vi "Drag Start Row Visualization.vi"(7 "DragStart? (F)":bool, 8 "error in (no error)":errorcluster, 10 "DragStart Indices":i32[](array[numeric]), 11 "BetterListboxHandle in":refnum<class "BetterListboxHandle.lvclass">) -> (0 "error out":errorcluster, 3 "BetterListboxHandle out":refnum<class "BetterListboxHandle.lvclass">)   [LabVIEW 2020, in "BetterDragAndDrop.lvlib" / "BetterListboxHandle.lvclass"]
uses:
  BetterListboxHandle.lvclass
  BetterListboxHandle.lvclass/BetterListboxHandle.ctl
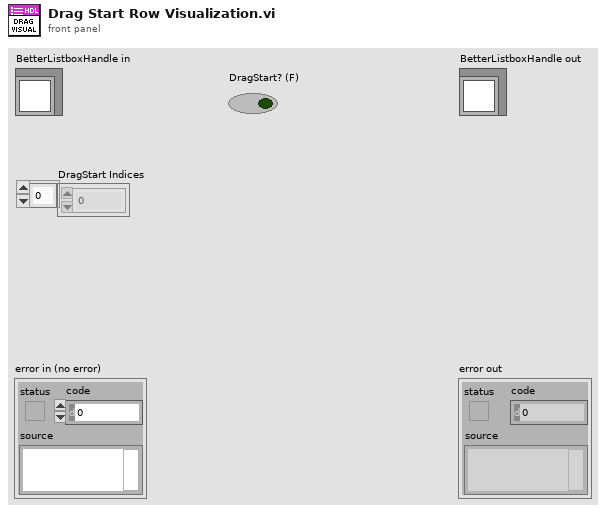
[diagram p1: front panel]
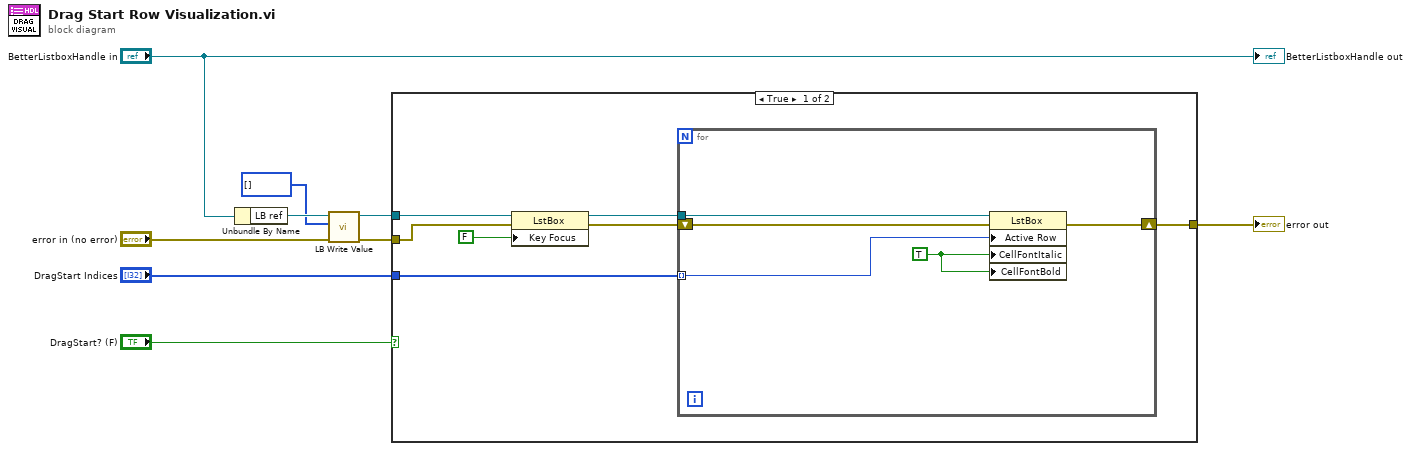
[diagram p0: block diagram]
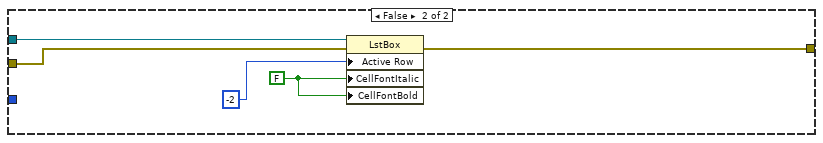
[diagram p2: hidden frame]
diagram:
  n1 = Unbundle By Name("BetterListboxHandle in") -> ("LB ref"=w8:refnum<vi>)
  n2 = call "LB Write Value.vi"("error in (no error)"="error in (no error)", "Value"=i32[] [], "LB ref (generic)"=w8) -> ("error out"=w5:errorcluster, "LB ref (generic)"=w7:refnum<vi>)  [unwired: 7 in]
  n3 = case shown="True" "DragStart? (F)" {
    tunnel: w7 -> [w16 w25]
    tunnel: "DragStart Indices" -> [w13 _]
    tunnel: w5 -> [w11 w24]
    tunnel: [w10 w23] -> w1
    frame True {
      n4 = property class="LstBox"(reference=w16, error in=w11, "Key Focus"=FALSE) -> (reference out=w14:refnum<vi>, error out=w12:errorcluster)
      n5 = for {
        tunnel: w14 -> [w21]
        tunnel: w13 -> [w17] mode=indexing
        shift-right: [w18] -> w10
        shift-left: w12 -> [w19]
        w20 = TRUE ("Active Cell:Cell Font:Italic")
        n6 = property class="LstBox"(reference=w21, error in=w19, "Active Row"=w17, "CellFontItalic"=w20, "CellFontBold"=w20) -> (error out=w18:errorcluster)  [unwired: 1 out]
      }
    }
    frame False {
      w26 = FALSE ("Active Cell:Cell Font:Italic")
      n7 = property class="LstBox"(reference=w25, error in=w24, "Active Row"=-2 ("Row"), "CellFontItalic"=w26, "CellFontBold"=w26) -> (error out=w23:errorcluster)  [unwired: 1 out]
    }
  }
  "error out" <- w1
  "BetterListboxHandle out" <- "BetterListboxHandle in"
